vi "labview_visualization.vi"() -> ()   [LabVIEW 2016]
uses:
  <vilib>/Instr/_visa.llb/VISA Configure Serial Port (Instr).vi
panel:
  out "Roll":dbl(graph)
  out "Pitch":dbl(graph)
  out "Yaw":dbl(graph)
  out "Roll":dbl
  out "Pitch":dbl
  out "Yaw":dbl
  in  "baud rate (9600)":u32=9600
  out "Roll":dbl(knob) scale=-180.0..180.0
  out "Pitch":dbl(knob) scale=-180.0..180.0
  out "Yaw":dbl(knob) scale=-180.0..180.0
  in  "VISA resource name":refnum<visa-resource-name>
  in  "stop":bool
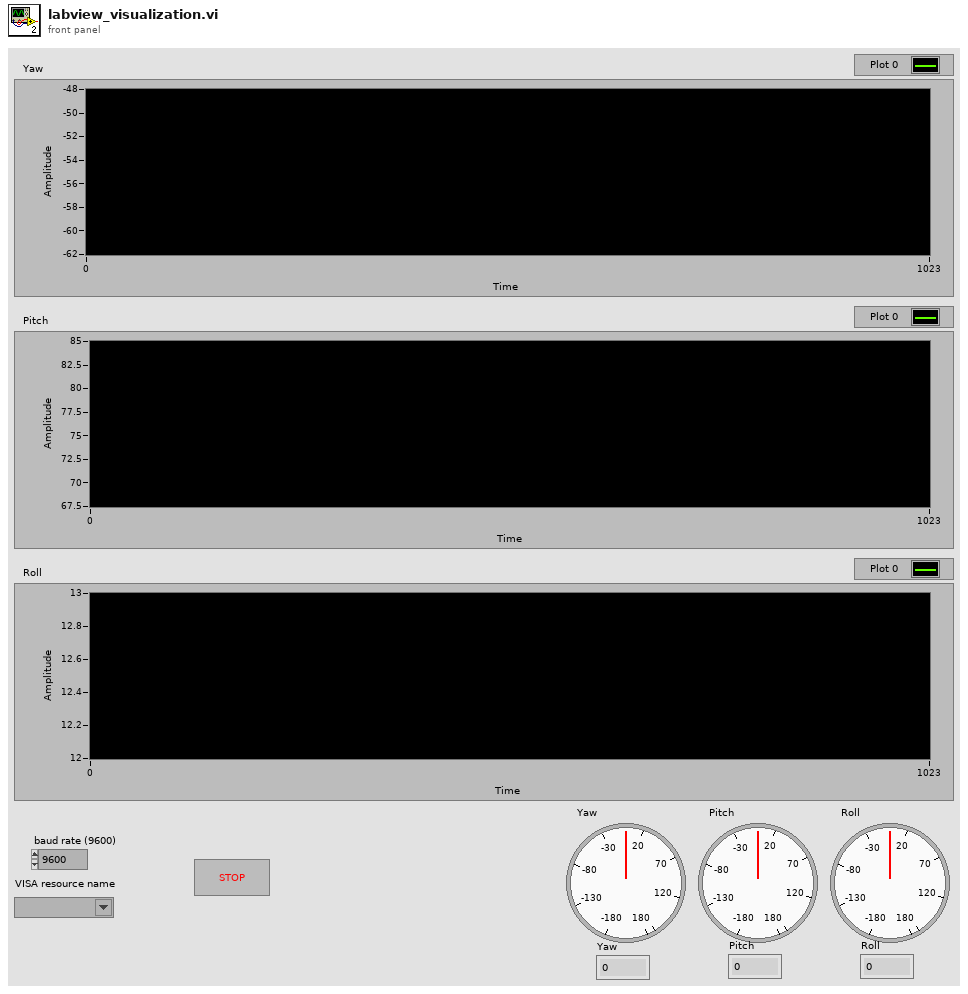
[diagram p1: front panel]
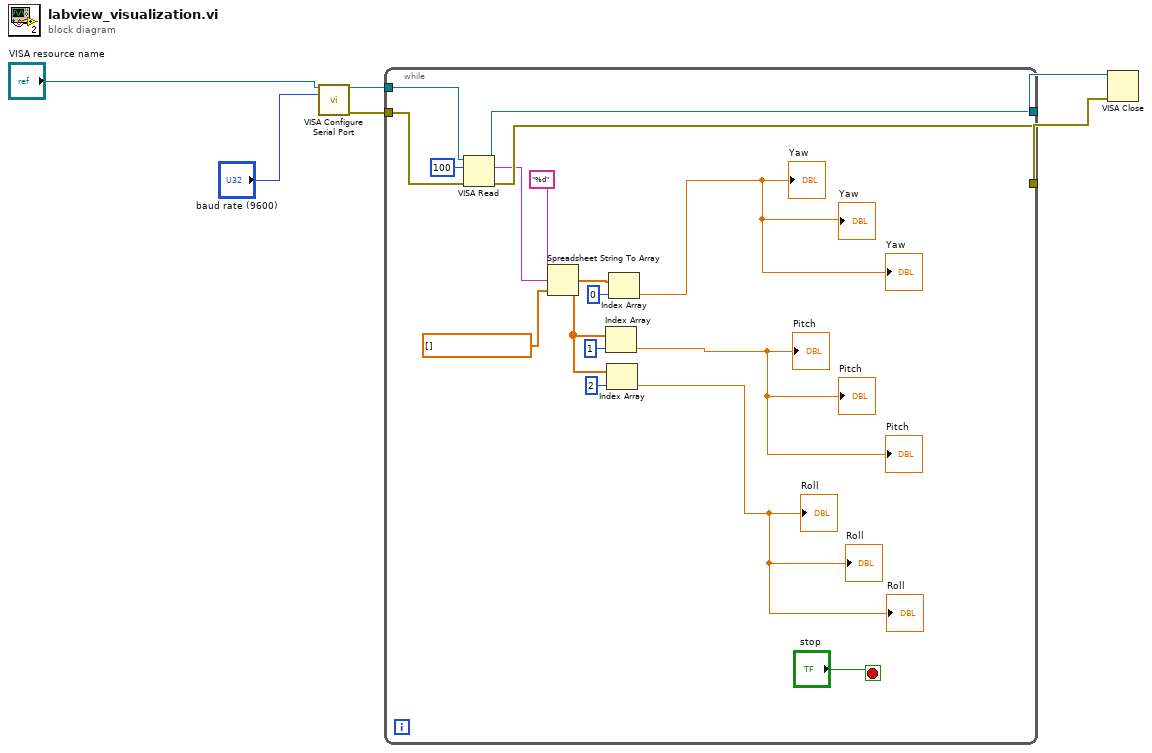
[diagram p0: block diagram]
diagram:
  n1 = call-poly "VISA Configure Serial Port"("VISA resource name"="VISA resource name", "baud rate (9600)"="baud rate (9600)") -> ("VISA resource name out"=w4:refnum<visa-resource-name>, "error out"=w3:errorcluster)  [unwired: 12 in]
  n2 = while {
    tunnel: [w21] -> w6
    tunnel: [w20] -> w5
    tunnel: w4 -> [w19]
    tunnel: w3 -> [w18]
    stop <- "stop" stop-if-true
    n3 = VISA Read(VISA resource name=w19, byte count=u32 100, error in (no error)=w18) -> (VISA resource name out=w21:refnum<visa-resource-name>, read buffer=w10:string, error out=w20:errorcluster)  [unwired: 1 out]
    n4 = Spreadsheet String To Array(format string="%d", spreadsheet string=w10, array type (2D Dbl)=dbl[] []) -> (array=w11:dbl[])  [unwired: 1 in]
    n5 = Index Array(array=w11, index=1) -> (element=→"Pitch" →"Pitch" →"Pitch":dbl)
    n6 = Index Array(array=w11, index=2) -> (element=→"Roll" →"Roll" →"Roll":dbl)
    n7 = Index Array(array=w11, index=0) -> (element=→"Yaw" →"Yaw" →"Yaw":dbl)
  }
  n8 = VISA Close(VISA resource name=w6, error in (no error)=w5) -> ()  [unwired: 1 out]
